vi "Rename Alias.vi"(8 "error in":errorcluster, 9 "new alias name":string, 10 "alias":string, 11 "endpoint aliases in":T1 format="%.0x") -> (0 "error out":errorcluster, 3 "endpoint aliases out":T1 format="%.0x")   [LabVIEW 2017, in "Routing and Faulting Scripting.lvlib"]
uses:
  Routing and Faulting Scripting.lvlib
  <vilib>/NI Veristand/Custom Device API/Custom Device Item Ref.ctl
  <vilib>/NI Veristand/Custom Device API/Custom Device API.lvlib
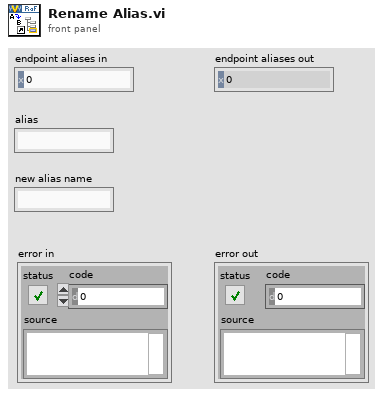
[diagram p1: front panel]
types:
  T1 = typedef "Custom Device API.lvlib/Custom Device Item Ref.ctl" = u64
  T2 = typedef "Routing and Faulting Shared.lvlib/Alias Endpoint.ctl" = cluster{"Module Path":string, "Endpoint":string}
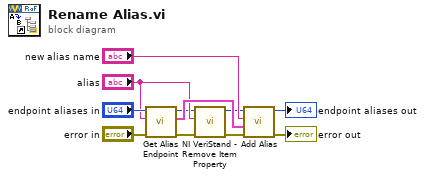
[diagram p0: block diagram]
diagram:
  n1 = call "Get Alias Endpoint.vi"("error in"="error in", "alias"="alias", "endpoint aliases in"="endpoint aliases in") -> ("error out"=w5:errorcluster, "endpoint"=w9:T2, "endpoint aliases out"=w6:T1)  [unwired: 6 in]
  n2 = call <vilib>:"NI VeriStand - Remove Item Property.vi"("error in (no error)"=w5, "Property Name"="alias", "Item Ref in"=w6) -> ("error out"=w3:errorcluster, "Item Ref out"=w4:T1)  [unwired: 6 in, 1 out]
  n3 = call "Add Alias.vi"("error in"=w3, "endpoint"=w9, "alias"="new alias name", "endpoint aliases in"=w4) -> ("error out"=→"error out":errorcluster, "endpoint aliases out"=→"endpoint aliases out":T1)  [unwired: 6 in]
